vi "Perform_Meas_Setup.vi"(2 "Simulate/Run":T1, 3 "String array":string[](array[string])) -> (0 "Continue?":bool)   [LabVIEW 2011]
uses:
  Controls/User_Specific_mode.ctl
  Controls/Save_Data.ctl
  Controls/Setup.ctl
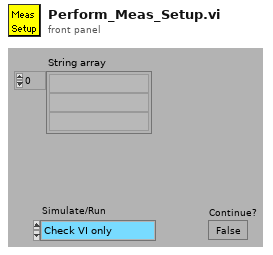
[diagram p1: front panel]
types:
  T1 = typedef "User_Specific_mode.ctl" = enum16{"Check VI only", "Run VI"}
  T2 = typedef "Save_Data.ctl" = enum16{"Save No Data", "Save Data"}
  T3 = typedef "Setup.ctl" = enum16{"Run Program", "Show Setup", "Save Current Setup", "Setup Front Panel"}
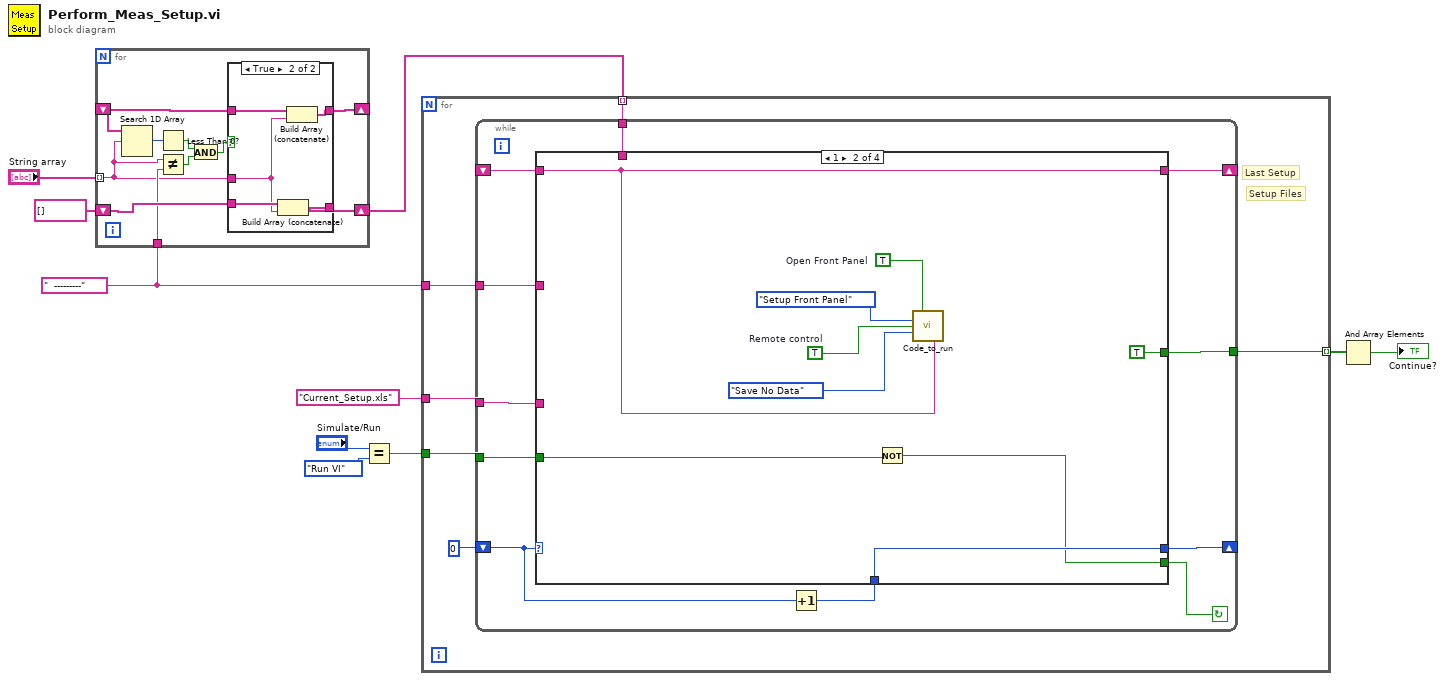
[diagram p0: block diagram]
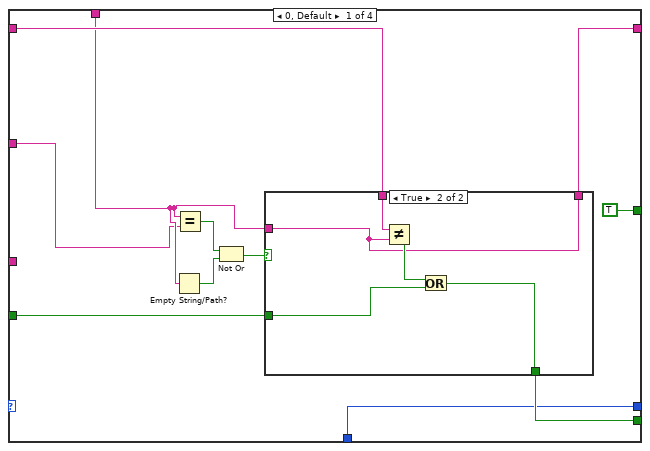
[diagram p3: hidden frame]
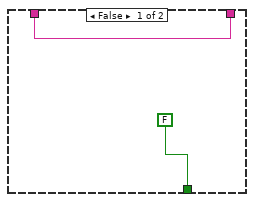
[diagram p4: hidden frame]
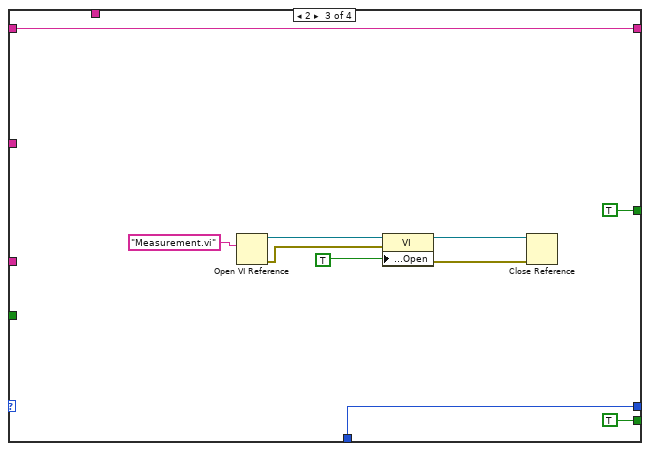
[diagram p5: hidden frame]
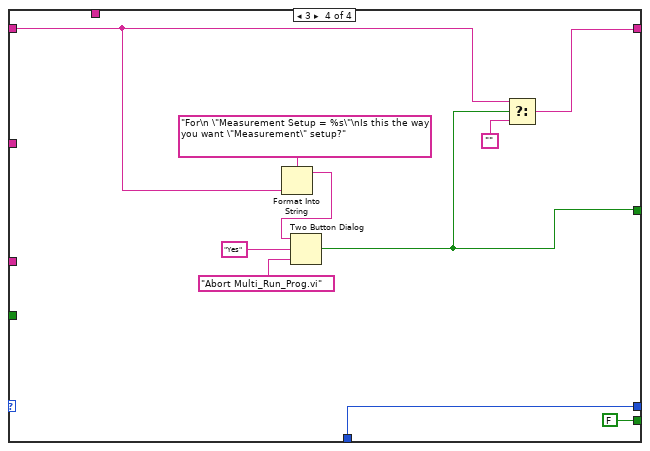
[diagram p6: hidden frame]
diagram:
  w1 = "  ---------" ("f")
  n1 = for {
    shift-right: [w19] -> _
    shift-left: _ -> [w20]
    shift-right: [w17] -> w2
    shift-left: string[] [] -> [w18]
    tunnel: "String array" -> [w14] mode=indexing
    tunnel: w1 -> [w15]
    n2 = Search 1D Array(1D array=w20, element=w14) -> (index of element=w16:i32)  [unwired: 1 in]
    n3 = Less Than 0?(x=w16) -> (x < 0?=w11:bool)
    n4 = Not Equal?(x=w14, y=w15) -> (x != y?=w12:bool)
    n5 = And(x=w11, y=w12) -> (x .and. y?=w13:bool)
    n6 = case shown="True" w13 {
      tunnel: w14 -> [_ w23]
      tunnel: w20 -> [w22 w27]
      tunnel: [w22 w26] -> w19
      tunnel: w18 -> [w21 w25]
      tunnel: [w21 w24] -> w17
      frame False {
      }
      frame True {
        n7 = Build Array (concatenate)(w25, w23) -> (w24:string[])
        n8 = Build Array (concatenate)(w27, w23) -> (w26:string[])
      }
    }
  }
  n9 = Equal?(x="Simulate/Run", y=User_Specific_mode."Run VI" ("Simulate/Run")) -> (x = y?=w7:bool)
  n10 = for {
    tunnel: "Current_Setup.xls" ("name or relative path") -> [w32]
    tunnel: w7 -> [w31]
    tunnel: w2 -> [w30] mode=indexing
    tunnel: [w29] -> w6 mode=indexing
    tunnel: w1 -> [w28]
    # "Last Setup"
    # "Setup Files"
    n11 = while {
      tunnel: w31 -> [w36]
      tunnel: w32 -> [w37]
      shift-left: _ -> [w39]
      shift-right: [w38] -> _
      tunnel: [w40] -> w29
      shift-left: 0 -> [w43]
      shift-right: [w41] -> _
      tunnel: w30 -> [w35]
      tunnel: w28 -> [w34]
      stop <- w44 continue-if-true
      n12 = Increment(x=w43) -> (x+1=w42:i32)
      n13 = case shown="1" w43 {
        tunnel: [w52 w66 TRUE FALSE] -> w44
        tunnel: w42 -> [w50 w68 w81 w91]
        tunnel: [w50 w68 w81 w91] -> w41
        tunnel: [TRUE ("T button?") TRUE ("T button?") TRUE ("T button?") w85] -> w40
        tunnel: w39 -> [w54 w63 w80 w83]
        tunnel: [w53 w63 w80 w84] -> w38
        tunnel: w37 -> [_ _ _ _]
        tunnel: w36 -> [w51 w67 _ _]
        tunnel: w35 -> [w46 _ _ _]
        tunnel: w34 -> [w45 _ _ _]
        frame 0, Default {
          n14 = Empty String/Path?(string/path=w46) -> (empty?=w48:bool)
          n15 = Equal?(x=w46, y=w45) -> (x = y?=w49:bool)
          n16 = Not Or(1:w48, 2:w49) -> (0:w47:bool)
          n17 = case shown="True" w47 {
            tunnel: [w57 w59] -> w53
            tunnel: w46 -> [_ w59]
            tunnel: w54 -> [w57 w62]
            tunnel: [FALSE w60] -> w52
            tunnel: w51 -> [_ w58]
            frame False {
            }
            frame True {
              n18 = Not Equal?(x=w62, y=w59) -> (x != y?=w61:bool)
              n19 = Or(x=w61, y=w58) -> (x .or. y?=w60:bool)
            }
          }
        }
        frame 1 {
          w70 = TRUE  # Remote control
          w71 = TRUE  # Open Front Panel
          n20 = Not(x=w67) -> (.not. x?=w66:bool)
          n21 = call "Code_to_run.vi"("Open Front Panel"=w71, "setup"=Setup."Setup Front Panel", "Remote control"=w70, "File"=Save_Data."Save No Data", "Setup filename"=w63) -> ()  [unwired: 5 in, 6 out]
        }
        frame 2 {
          n22 = Open VI Reference(vi path="Measurement.vi") -> (vi reference=w76:refnum<vi>, error out=w77:errorcluster)  [unwired: 1 in, 4 out]
          n23 = property class="VI"(reference=w76, error in=w77, "Front Panel Window:Open"=TRUE) -> (reference out=w74:refnum<vi>, error out=w73:errorcluster)
          n24 = Close Reference(reference=w74, error in (no error)=w73) -> ()  [unwired: 1 out]
        }
        frame 3 {
          n25 = Format Into String(format string="For\n \"Measurement Setup = %s\"\nIs this the way you want \"Measurement\" setup?" ("message"), w83) -> (resulting string=w90:string)  [unwired: 2 in, 1 out]
          n26 = Two Button Dialog(message=w90, 1:"Abort Multi_Run_Prog.vi" ("F button name (\"Cancel\")"), 2:"Yes" ("T button name (\"OK\")")) -> (T button?=w85:bool)
          n27 = Select(t=w83, s=w85, f="") -> (s? t:f=w84:string)
        }
      }
    }
  }
  n28 = And Array Elements(Boolean array=w6) -> (logical AND=→"Continue?":bool)
